vi "Random Number.vi"(1 "Min":dbl, 2 "Max":dbl) -> (0 "Out":dbl)   [LabVIEW 2010]
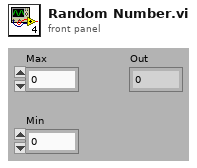
[diagram p1: front panel]
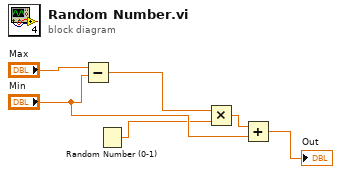
[diagram p0: block diagram]
diagram:
  n1 = Subtract(x="Max", y="Min") -> (x-y=w2:dbl)
  n2 = Random Number (0-1)() -> (number: 0 to 1=w3:dbl)
  n3 = Multiply(x=w2, y=w3) -> (x*y=w4:dbl)
  n4 = Add(x=w4, y="Min") -> (x+y=→"Out":dbl)
